vi "QDM matlab saver_101freqs_rt.vi"(3 "NumofFreq":dbl, 4 "numFreqs":i32=101, 6 "img data stack Input":dbl[][](array[numeric]), 7 "matlab path":path, 8 "Height":i64(slide)=1200 min=0 max=1200 step=4 scale=0.0..1200.0, 9 "Width":i64(slide)=1920 min=0 max=1920 step=4 scale=0.0..1920.0, 10 "freq list (Hz)":dbl[](array[numeric]), 11 "sweep #":i32) -> ()   [LabVIEW 2019]
panel:
  out "NumofFreq 2":i32=101
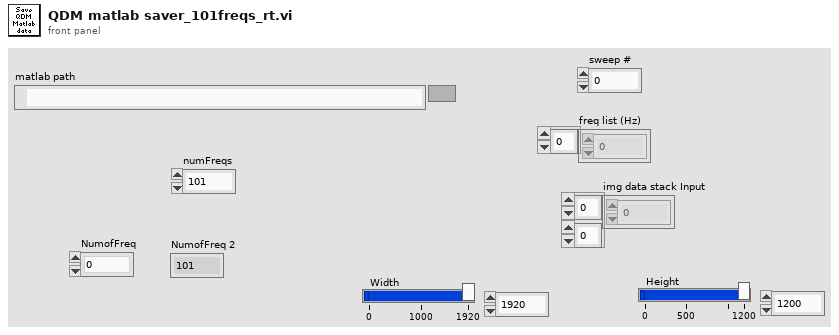
[diagram p1: front panel]
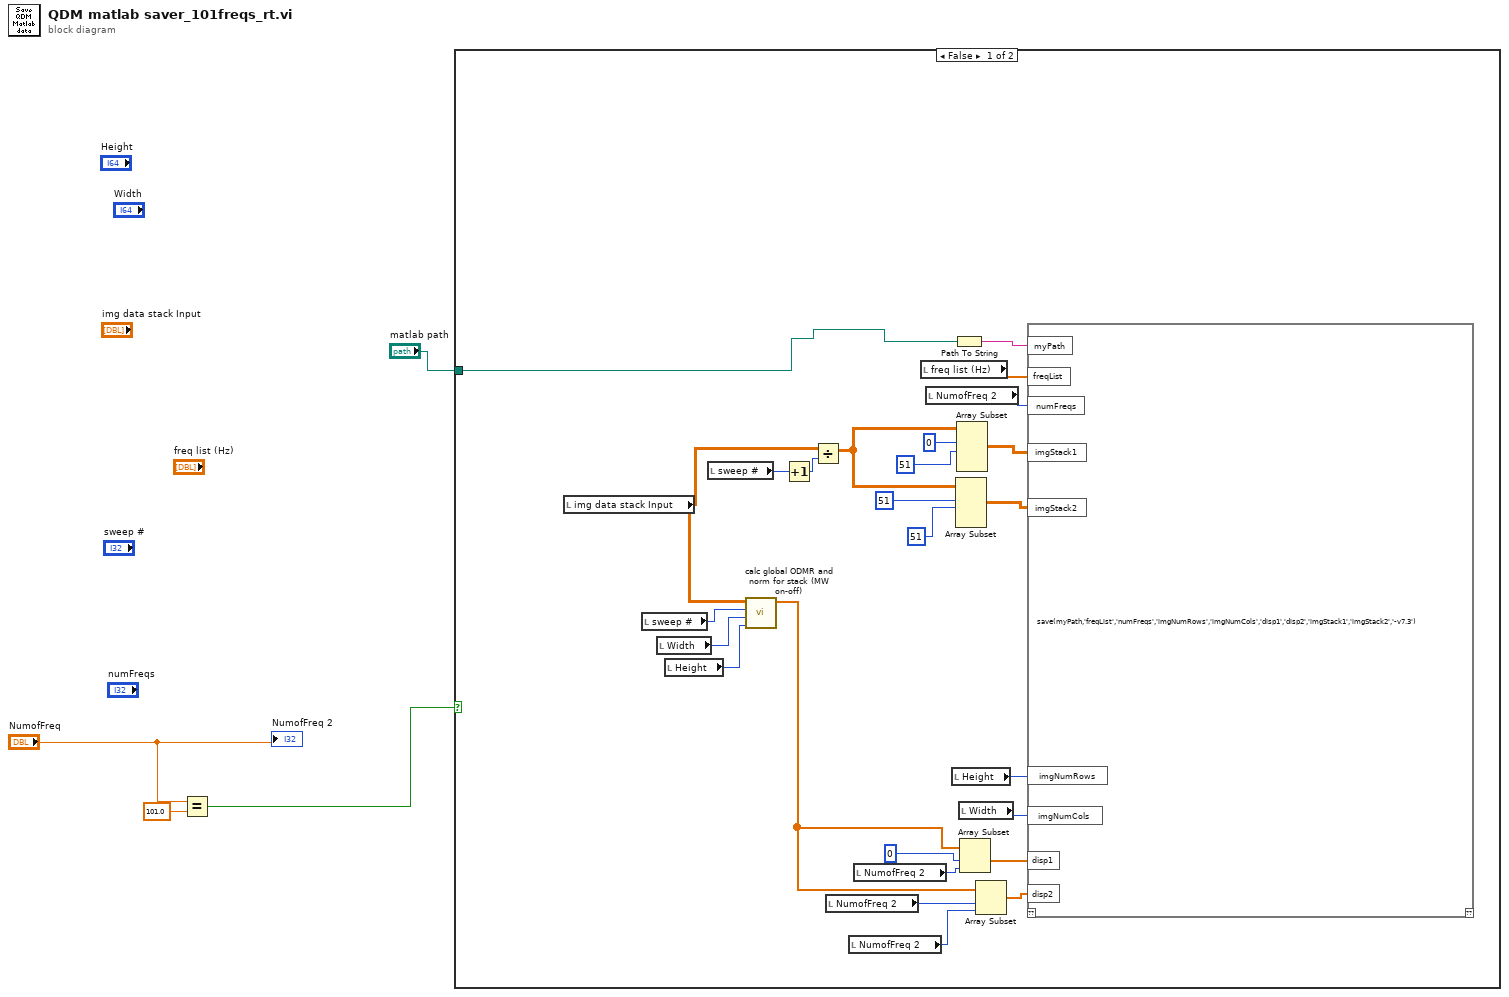
[diagram p0: block diagram]
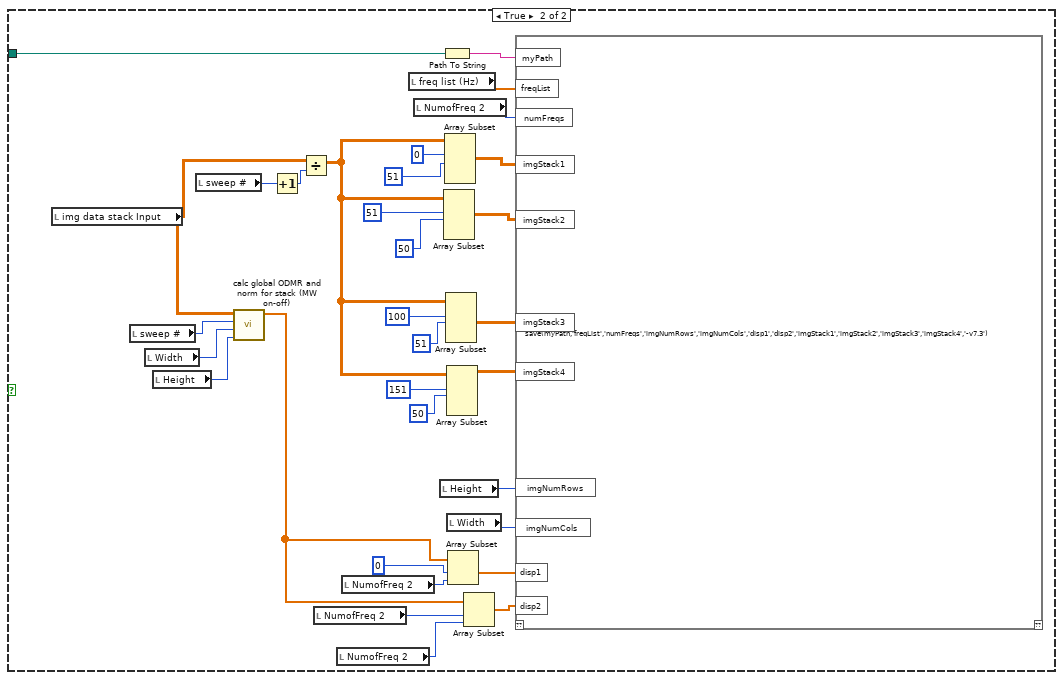
[diagram p2: hidden frame]
diagram:
  n1 = Equal?(x="NumofFreq", y=101.0) -> (x = y?=w2:bool)
  n2 = case shown="False" w2 {
    tunnel: "matlab path" -> [w5 w31]
    frame False {
      n3 = local read "img data stack Input"() -> (w12:dbl[][])
      n4 = local read "sweep #"() -> (w13:i32)
      n5 = local read "Width"() -> (w17:i64)
      n6 = local read "Height"() -> (w18:i64)
      n7 = local read "sweep #"() -> (w15:i32)
      n8 = call "calc global ODMR and norm for stack (MW on-off).vi"("Height"=w18, "Width"=w17, "sweep #"=w13, "img data stack"=w12) -> ("normed spectrum"=w16:dbl[])  [unwired: 7 in]
      n9 = Increment(x=w15) -> (x+1=w14:i32)
      n10 = Divide(x=w12, y=w14) -> (x/y=w11:dbl[][])
      n11 = local read "NumofFreq 2"() -> (w24:i32)
      n12 = local read "NumofFreq 2"() -> (w23:i32)
      n13 = local read "NumofFreq 2"() -> (w25:i32)
      n14 = local read "freq list (Hz)"() -> (w29:dbl[])
      n15 = local read "NumofFreq 2"() -> (w28:i32)
      n16 = local read "Height"() -> (w26:i64)
      n17 = Path To String(path=w5) -> (string=w30:string)
      n18 = Array Subset(array=w11, index (row)=51, length (row)=51) -> (w19:dbl[][])  [unwired: 2 in]
      n19 = Array Subset(array=w11, index (row)=0 ("index"), length (row)=51) -> (w20:dbl[][])  [unwired: 2 in]
      n20 = local read "Width"() -> (w27:i64)
      n21 = Array Subset(array=w16, index=0, length=w25) -> (w22:dbl[])
      n22 = Array Subset(array=w16, index=w24, length=w23) -> (w21:dbl[])
      n23 = script code="save(myPath,'freqList','numFreqs','imgNumRows','imgNumCols','disp1','disp2','imgStack1','imgStack2','-v7.3')"("myPath"=w30, "freqList"=w29, "imgStack1"=w20, "numFreqs"=w28, "imgNumRows"=w26, "imgNumCols"=w27, "disp1"=w22, "disp2"=w21, "imgStack2"=w19) -> ()  [unwired: 1 in, 1 out]
    }
    frame True {
      n24 = local read "img data stack Input"() -> (w59:dbl[][])
      n25 = local read "sweep #"() -> (w58:i32)
      n26 = local read "Width"() -> (w54:i64)
      n27 = local read "Height"() -> (w53:i64)
      n28 = local read "sweep #"() -> (w56:i32)
      n29 = call "calc global ODMR and norm for stack (MW on-off).vi"("Height"=w53, "Width"=w54, "sweep #"=w58, "img data stack"=w59) -> ("normed spectrum"=w55:dbl[])  [unwired: 7 in]
      n30 = Increment(x=w56) -> (x+1=w57:i32)
      n31 = Divide(x=w59, y=w57) -> (x/y=w60:dbl[][])
      n32 = local read "NumofFreq 2"() -> (w47:i32)
      n33 = local read "NumofFreq 2"() -> (w48:i32)
      n34 = local read "NumofFreq 2"() -> (w46:i32)
      n35 = local read "freq list (Hz)"() -> (w42:dbl[])
      n36 = local read "NumofFreq 2"() -> (w43:i32)
      n37 = local read "Height"() -> (w45:i64)
      n38 = Path To String(path=w31) -> (string=w41:string)
      n39 = Array Subset(array=w60, index (row)=51, length (row)=50) -> (w52:dbl[][])  [unwired: 2 in]
      n40 = Array Subset(array=w60, index (row)=0 ("index"), length (row)=51) -> (w51:dbl[][])  [unwired: 2 in]
      n41 = Array Subset(array=w60, index (row)=100, length (row)=51) -> (w61:dbl[][])  [unwired: 2 in]
      n42 = Array Subset(array=w60, index (row)=151, length (row)=50) -> (w62:dbl[][])  [unwired: 2 in]
      n43 = local read "Width"() -> (w44:i64)
      n44 = Array Subset(array=w55, index=0, length=w46) -> (w49:dbl[])
      n45 = Array Subset(array=w55, index=w47, length=w48) -> (w50:dbl[])
      n46 = script code="save(myPath,'freqList','numFreqs','imgNumRows','imgNumCols','disp1','disp2','imgStack1','imgStack2','imgStack3','imgStack4','-v7.3')"("myPath"=w41, "freqList"=w42, "imgStack1"=w51, "numFreqs"=w43, "imgNumRows"=w45, "imgNumCols"=w44, "disp1"=w49, "disp2"=w50, "imgStack2"=w52, "imgStack3"=w61, "imgStack4"=w62) -> ()  [unwired: 1 in, 1 out]
    }
  }
  "NumofFreq 2" <- "NumofFreq"
